vi "Create command queue.vi"(8 "error in (no error)":errorcluster) -> (0 "error out":errorcluster)   [LabVIEW 2020, in "queue_core_loop.lvlib"]
uses:
  queue_core_loop.lvlib
  PTRL/dev_and_debug_tools/QueueMessage typedef.ctl
  PTRL/dev_and_debug_tools/dev_and_debug_tools.lvlib
panel:
  # "Development\ncontrols/indicators useful for development and testing, but which are not outputs of the VI"
  # "Input\nInputs to the VI"
  # "Output\nOutputs of the VI"
  # "Description\n\nBlank VI with error handling case. \n\nSummarize the use of this VI in this space."
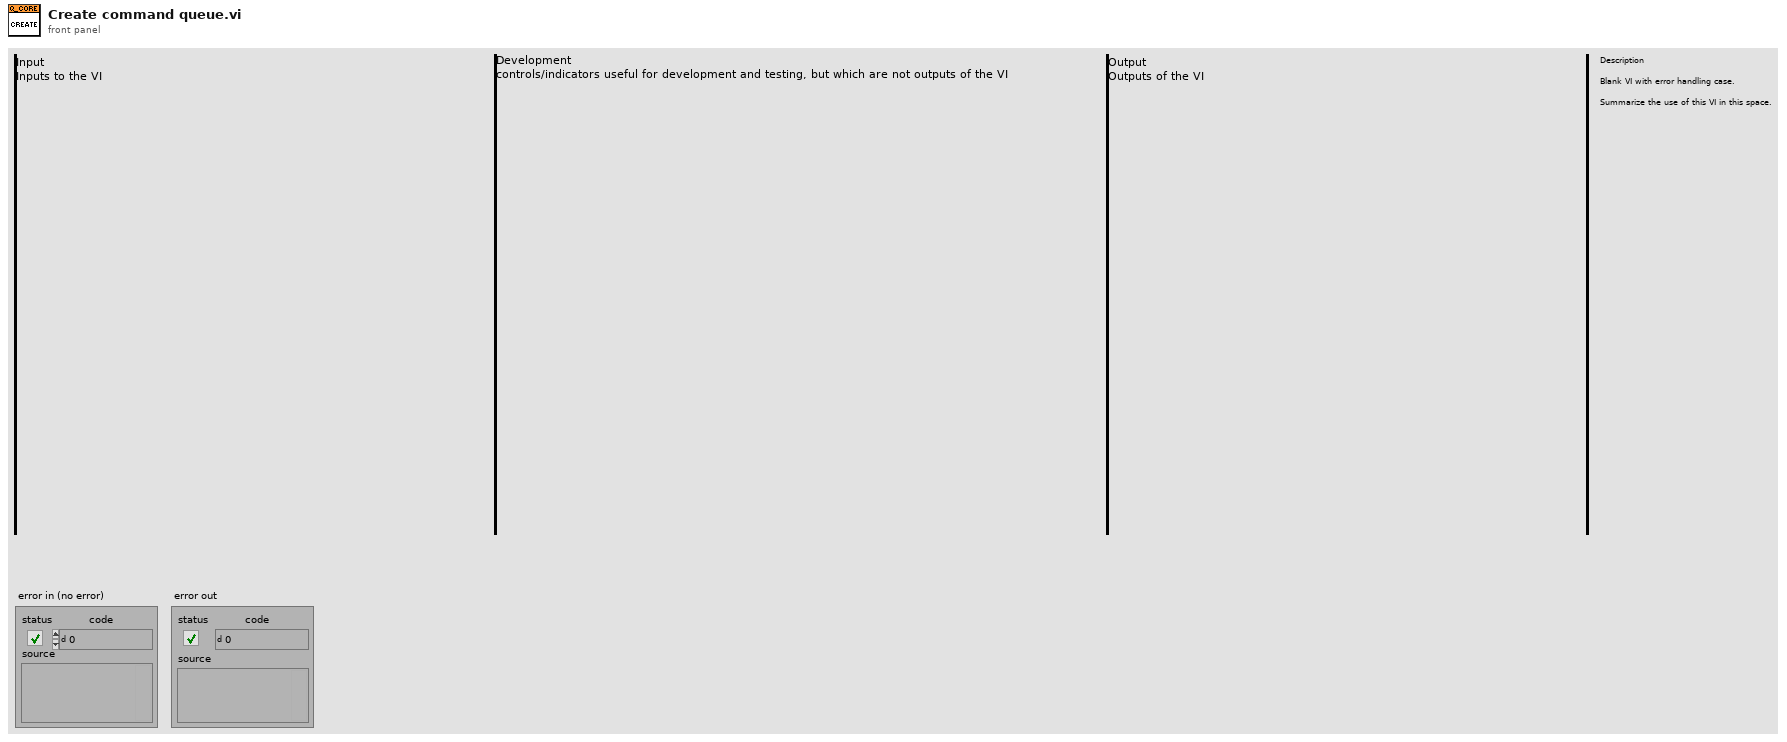
[diagram p1: front panel]
types:
  T1 = typedef "dev_and_debug_tools.lvlib/QueueMessage typedef.ctl" = cluster{"command":string, "data":variant}
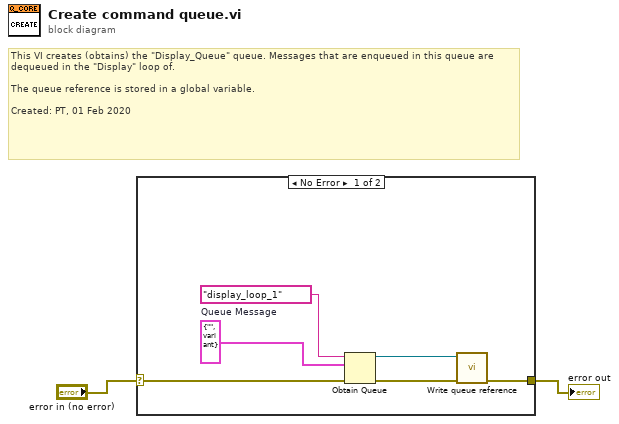
[diagram p0: block diagram]
diagram:
  # "This VI creates (obtains) the \"Display_Queue\" queue. Messages that are enqueued in this queue are dequeued in the \"Display\" loop of.\n\nThe queue reference is stored in a global variable.\n\nCreated: PT, 01 Feb 2020"
  n1 = case shown="No Error" "error in (no error)" {
    selector: "error in (no error)" -> [w8 w9]
    tunnel: [w3 w9] -> w1
    frame No Error {
      w7 = T1 {"command"="", "data"=variant}  # Queue Message
      n2 = Obtain Queue(name (unnamed)="display_loop_1", element data type=w7, error in (no error)=w8) -> (queue out=w5:refnum<queue>, error out=w4:errorcluster)  [unwired: 2 in, 1 out]
      n3 = call "Write queue reference.vi"("error in (no error)"=w4, "ALA_Display_Queue ref"=w5) -> ("error out"=w3:errorcluster)  [unwired: 9 in]
    }
    frame Error {
    }
  }
  "error out" <- w1
